vi "error log tester.vi"() -> ()   [LabVIEW 2017]
uses:
  Logging/Error Log/Error log.ctl
  Global Variables/General Globals.vi
panel:
  out "queue name":string
  out "elements":T1[](array[typedef])
  out "max queue size":i32
  out "# elements in queue":i32
  in  "Add error":bool
  in  "Stop Button":bool
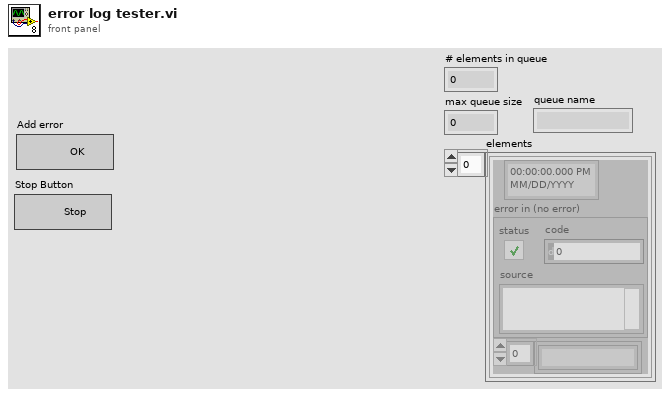
[diagram p1: front panel]
types:
  T1 = typedef "Error log.ctl" = cluster{timestamp, string[], "error in (no error)":errorcluster}
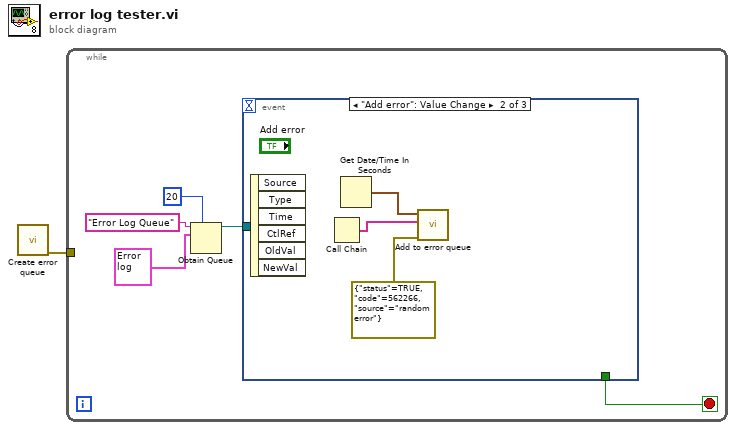
[diagram p0: block diagram]
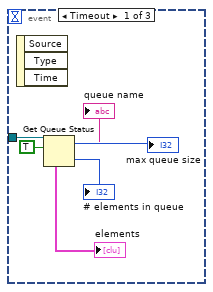
[diagram p2: hidden frame]
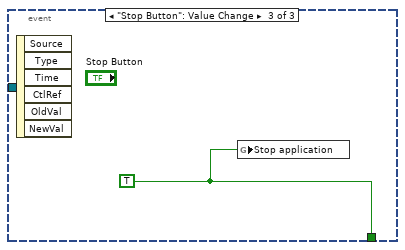
[diagram p3: hidden frame]
diagram:
  n1 = call "Create error queue.vi"() -> ("Error out"=w1:errorcluster)  [unwired: 11 in]
  n2 = while {
    tunnel: w1 -> [_]
    stop <- w6 stop-if-true
    n3 = Obtain Queue(max queue size (-1, unlimited)=20, name (unnamed)="Error Log Queue", element data type=T1 {timestamp(0 s since 1904-01-01), [], "error in (no error)"={"status"=FALSE, "code"=0, "source"=""}}) -> (queue out=w3:refnum<queue>)  [unwired: 2 in, 2 out]
    n4 = event shown="[1] \"Add error\": Value Change" {
      selector: _ -> [_ _ _]
      dyn-events: _ -> [_ _ _]
      timeout: _ -> [_ _ _]
      tunnel: [_ _ w16] -> w6
      tunnel: w3 -> [w10 _ _]
      event Timeout {
        n5 = event-data() -> ()  [unwired: 1 in, 3 out]
        n6 = Get Queue Status(queue=w10, return elements? (F)=TRUE) -> (queue name=→"queue name":string, max queue size=→"max queue size":i32, # elements in queue=→"# elements in queue":i32, elements=→"elements":T1[])  [unwired: 1 in, 4 out]
      }
      event "Add error": Value Change {
        n7 = event-data() -> ()  [unwired: 1 in, 6 out]
        n8 = Call Chain() -> (call chain=w14:string[])
        n9 = Get Date/Time In Seconds() -> (seconds since 1Jan1904=w15:timestamp)
        n10 = call "Add to error queue.vi"("error in (no error)"=errorcluster {"status"=TRUE, "code"=562266, "source"="random error"}, "Call Chain"=w14, "Time Stamp"=w15) -> ()  [unwired: 9 in]
      }
      event "Stop Button": Value Change {
        w16 = TRUE
        n11 = event-data() -> ()  [unwired: 1 in, 6 out]
        n12 = global write "General Globals.vi" "Stop application"(w16) -> ()
      }
    }
  }
